vi "loadICOSFiles.vi"(7 "working directory":path=path "c:/temp/ICOS", 11 "Path":string) -> ()   [LabVIEW 2012]
uses:
  <vilib>/addons/database/Connection.llb/DB Tools Open Connec (Path).vi
  <vilib>/addons/database/Connection.llb/Conn Execute.vi
  <vilib>/addons/database/Recordset.llb/Rec Fetch Recordset Data (R).vi
  <vilib>/addons/database/Recordset.llb/Rec Destroy - Connection.vi
  <vilib>/addons/database/_DB Variant To Data/Database Variant To Data.xnode
  <vilib>/addons/database/NI_Database_API.lvlib
panel:
  in  "working directory 2":path=path "c:/temp"
  out "error out":errorcluster
  out "concatenated string":string
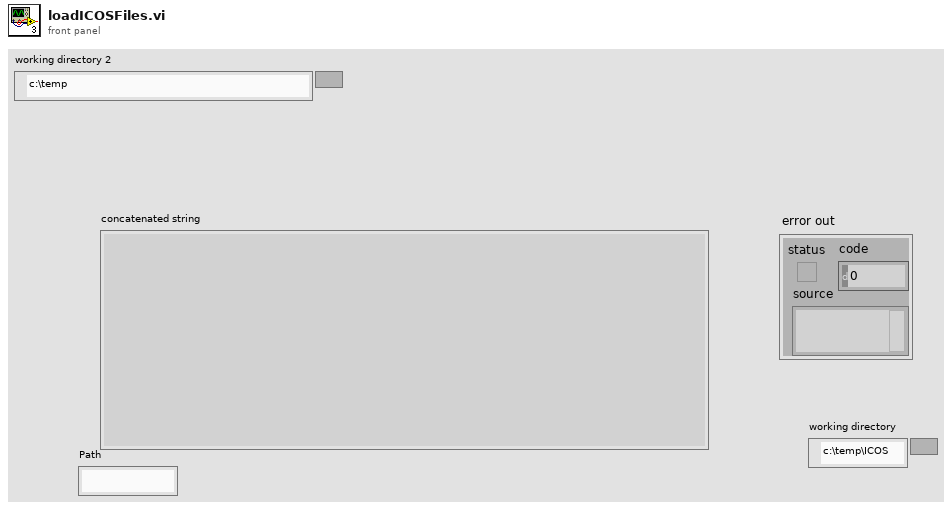
[diagram p1: front panel]
types:
  T1 = typedef "NI_Database_API.lvlib/Conn ObjectReference.ctl" = refnum<k1>
  T2 = typedef "NI_Database_API.lvlib/Rec ObjectReference.ctl" = refnum<k1>
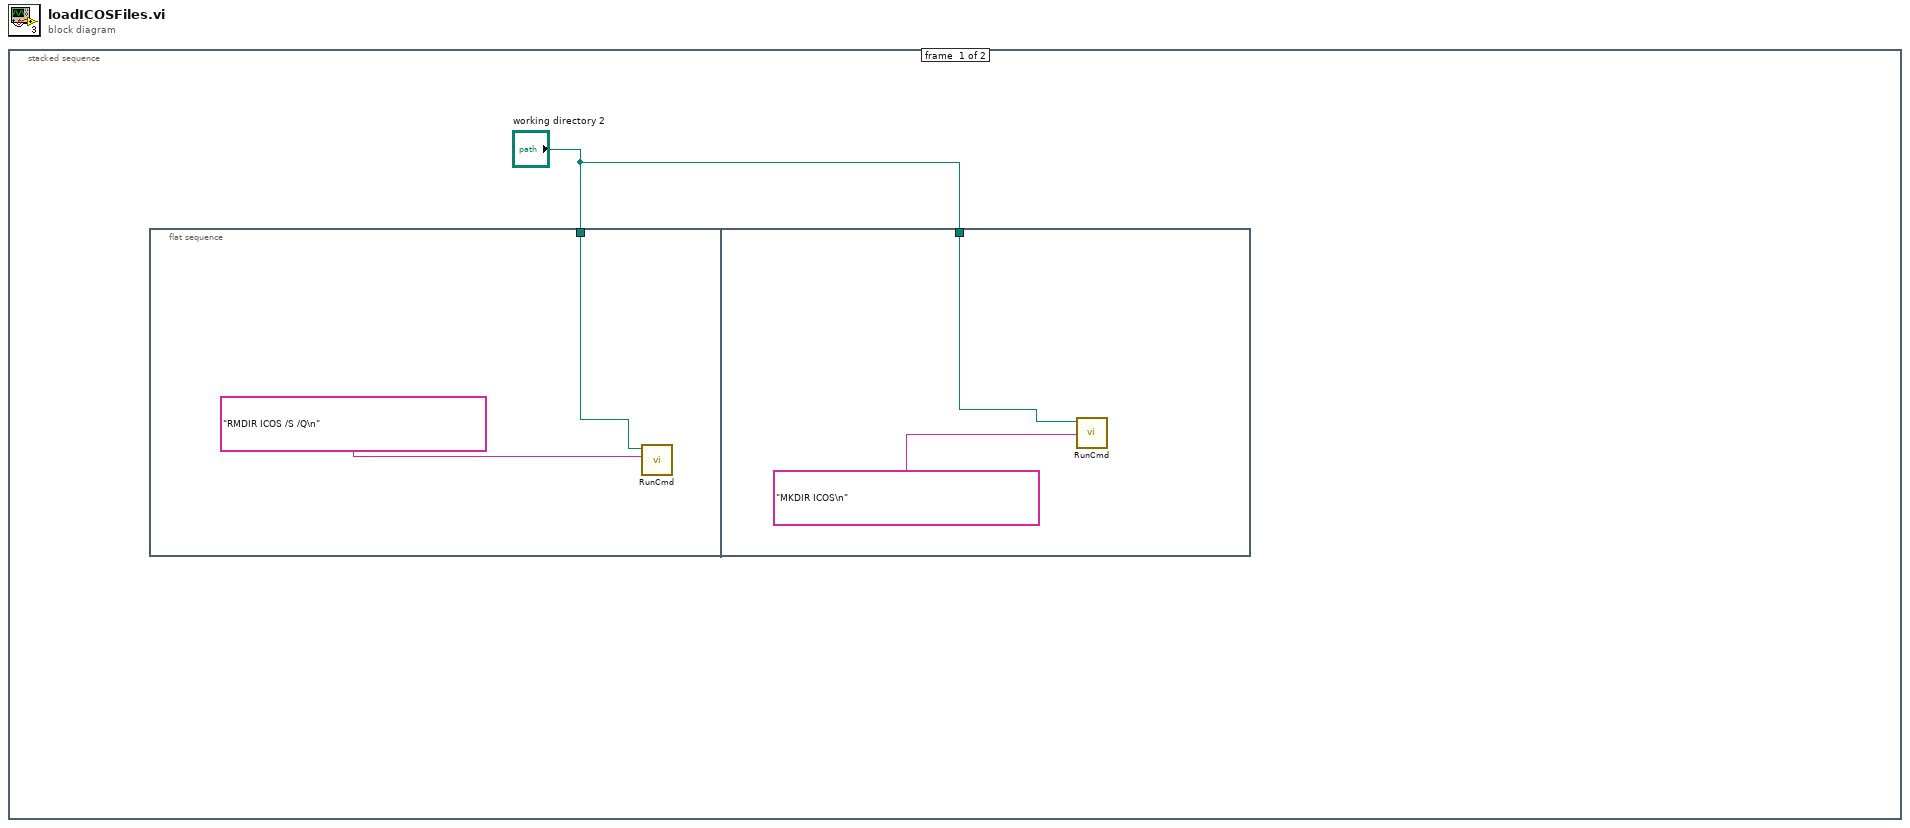
[diagram p0: block diagram]
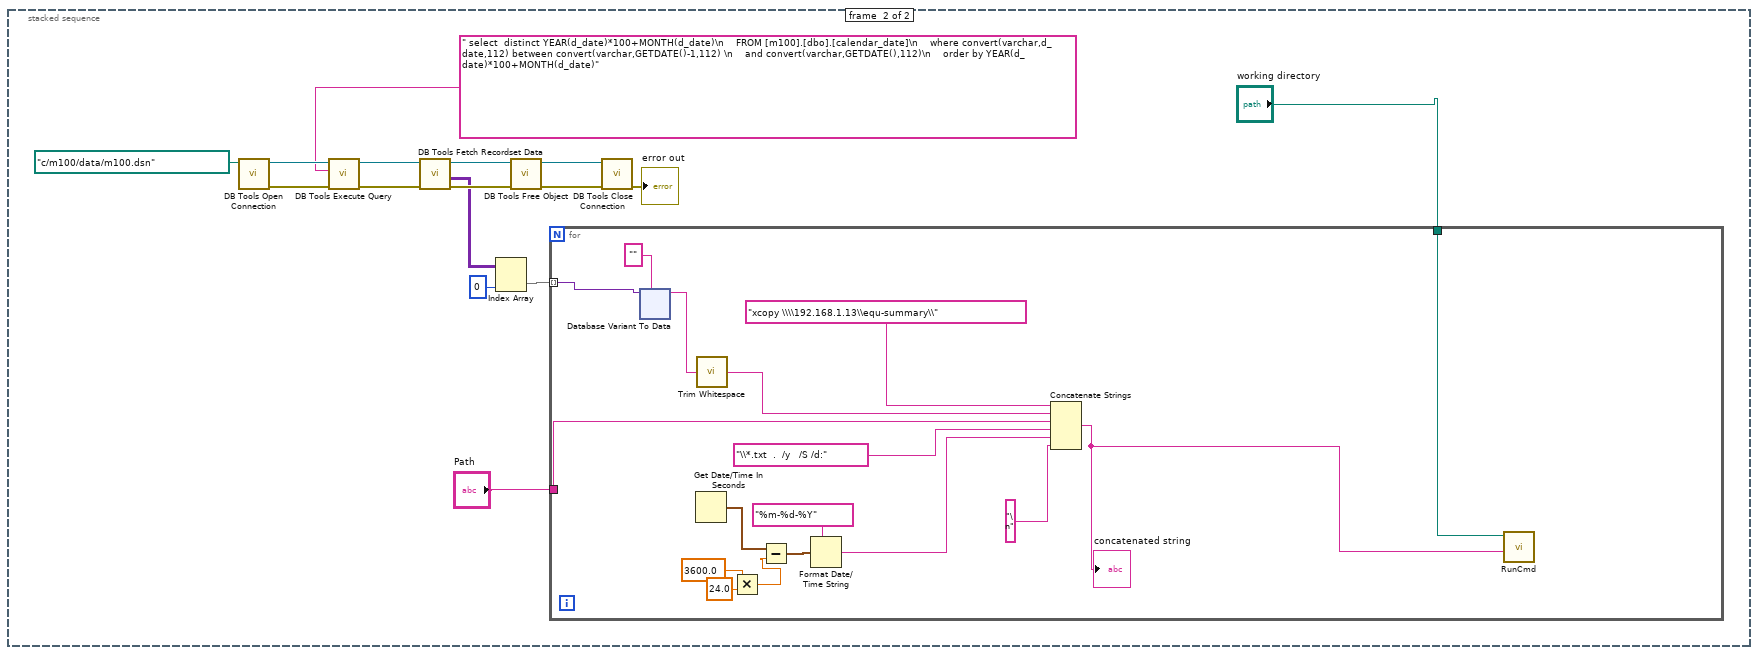
[diagram p2: hidden frame]
diagram:
  n1 = stacked-sequence {
    frame #0 {
      n2 = flat-sequence {
        tunnel: "working directory 2" -> [w2]
        tunnel: "working directory 2" -> [w4]
        frame #0 {
          n3 = call "RunCmd.vi"("Cmd String"="RMDIR ICOS /S /Q\n" ("standard input"), "working directory"=w2) -> ()  [unwired: 8 in, 2 out]
        }
        frame #1 {
          n4 = call "RunCmd.vi"("Cmd String"="MKDIR ICOS\n" ("standard input"), "working directory"=w4) -> ()  [unwired: 8 in, 2 out]
        }
      }
    }
    frame #1 {
      n5 = call-poly <vilib>:"DB Tools Open Connection.vi"("connection information"=path "c:/m100/data/m100.dsn") -> ("error out"=w17:errorcluster, "connection reference"=w21:T1)  [unwired: 7 in]
      n6 = call-poly <vilib>:"DB Tools Execute Query.vi"("error in (no error)"=w17, "SQL query"=" select  distinct YEAR(d_date)*100+MONTH(d_date)\n    FROM [m100].[dbo].[calendar_date]\n    where convert(varchar,d_date,112) between convert(varchar,GETDATE()-1,112) \n    and convert(varchar,GETDATE(),112)\n    order by YEAR(d_date)*100+MONTH(d_date)", "connection reference"=w21) -> ("error out"=w16:errorcluster, "recordset reference"=w20:T2)  [unwired: 5 in]
      n7 = call-poly <vilib>:"DB Tools Fetch Recordset Data.vi"("error in (no error)"=w16, "recordset reference"=w20) -> ("error out"=w15:errorcluster, "recordset data"=w10:variant[][], "recordset reference out"=w19:T2)  [unwired: 3 in]
      n8 = Index Array(array=w10, index (col)=0 ("disabled index (col)")) -> (element=w8:variant[])  [unwired: 1 in]
      n9 = call-poly <vilib>:"DB Tools Free Object.vi"("error in (no error)"=w15, "recordset reference"=w19) -> ("error out"=w14:errorcluster, "connection reference"=w18:T1)  [unwired: 8 in]
      n10 = for {
        tunnel: w8 -> [w38] mode=indexing
        tunnel: "Path" -> [w24]
        tunnel: "working directory" -> [w22]
        n11 = xnode "Database Variant To Data"("database variant"=w38, "type"="") -> ("data"=w28:string)  [unwired: 1 in, 1 out]
        n12 = Get Date/Time In Seconds() -> (seconds since 1Jan1904=w29:timestamp)
        n13 = call <vilib>:"Trim Whitespace.vi"("string"=w28) -> ("trimmed string"=w25:string)  [unwired: 1 in]
        n14 = Multiply(x=3600.0, y=24.0) -> (x*y=w31:dbl)
        n15 = Subtract(x=w29, y=w31) -> (x-y=w32:timestamp)
        n16 = Format Date/Time String(time format string (%c)="%m-%d-%Y", seconds (now)=w32) -> (date/time string=w34:string)  [unwired: 1 in]
        n17 = Concatenate Strings("xcopy \\\\192.168.1.13\\equ-summary\\" ("string"), w25, w24, "\\*.txt  .  /y   /S /d:" ("string"), w34, "\n" ("string")) -> (w23:string)
        "concatenated string" <- w23
        n18 = call "RunCmd.vi"("Cmd String"=w23, "working directory"=w22) -> ()  [unwired: 8 in, 2 out]
      }
      n19 = call <vilib>:"DB Tools Close Connection.vi"("error in (no error)"=w14, "connection reference"=w18) -> ("error out"=→"error out":errorcluster)  [unwired: 5 in]
    }
  }
